vi "dfd_One Point Notch Peak Filter Design.vi"(7 "filter type":enum16{"Notch", "Peak"}(ring), 9 "normalized BW":dbl format="%.2f", 10 "Ab [dB]":dbl format="%.2f", 11 "normalized f0":dbl format="%.2f") -> (1 "denominator":dbl[](array[numeric]) format="%.2f", 2 "numerator":dbl[](array[numeric]) format="%.2f")   [LabVIEW 2017, in "NI_DigFilter_Design.lvlib"]
uses:
  <vilib>/addons/Digital Filter Design/NI_DigFilter_Design.lvlib
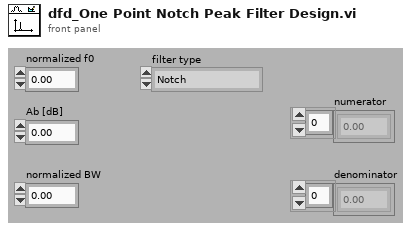
[diagram p1: front panel]
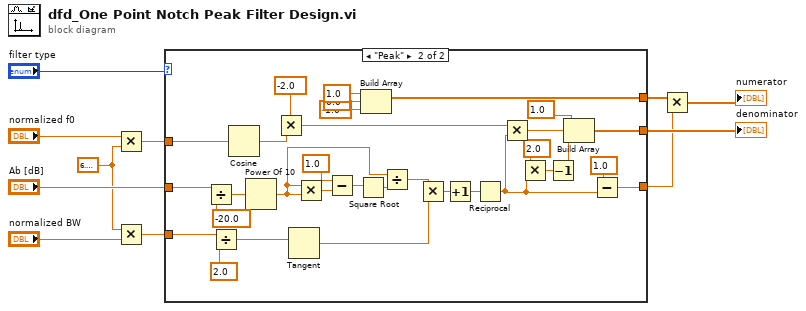
[diagram p0: block diagram]
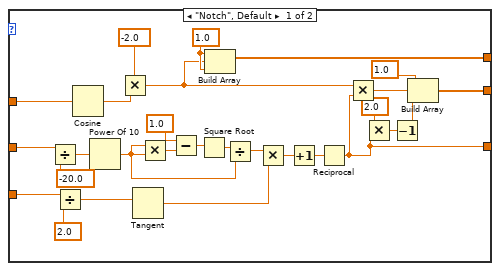
[diagram p2: hidden frame]
diagram:
  w3 = 6.283185307179586
  n1 = Multiply(x="normalized f0", y=w3) -> (x*y=w4:dbl)
  n2 = Multiply(x=w3, y="normalized BW") -> (x*y=w5:dbl)
  n3 = case shown="\"Peak\"" "filter type" {
    tunnel: "Ab [dB]" -> [w38 w70]
    tunnel: w5 -> [w34 w41]
    tunnel: [w21 w46] -> w6
    tunnel: w4 -> [w27 w40]
    tunnel: [w24 w60] -> w7
    tunnel: [w16 w54] -> w11
    frame "Notch", Default {
      w28 = 1.0 ("element")
      n4 = Divide(x=w38, y=-20.0) -> (x/y=w33:dbl)
      n5 = Divide(x=w34, y=2.0) -> (x/y=w29:dbl)
      n6 = Cosine(x=w27) -> (cos(x)=w26:dbl)
      n7 = Power Of 10(x=w33) -> (10^x=w35:dbl)
      n8 = Multiply(x=-2.0, y=w26) -> (x*y=w23:dbl)
      n9 = Tangent(1:w29) -> (0:w12:dbl)
      n10 = Multiply(x=w35, y=w35) -> (x*y=w37:dbl)
      n11 = Subtract(x=1.0, y=w37) -> (x-y=w15:dbl)
      n12 = Square Root(x=w15) -> (sqrt(x)=w14:dbl)
      n13 = Build Array(w28, w23, w28) -> (w24:dbl[])
      n14 = Divide(x=w14, y=w35) -> (x/y=w13:dbl)
      n15 = Multiply(x=w13, y=w12) -> (x*y=w31:dbl)
      n16 = Increment(x=w31) -> (x+1=w30:dbl)
      n17 = Reciprocal(x=w30) -> (1/x=w21:dbl)
      n18 = Multiply(x=w23, y=w21) -> (x*y=w22:dbl)
      n19 = Multiply(x=2.0 ("y"), y=w21) -> (x*y=w19:dbl)
      n20 = Decrement(x=w19) -> (x-1=w18:dbl)
      n21 = Build Array(1.0 ("element"), w22, w18) -> (w16:dbl[])
    }
    frame "Peak" {
      n22 = Divide(x=w70, y=-20.0) -> (x/y=w67:dbl)
      n23 = Divide(x=w41, y=2.0) -> (x/y=w63:dbl)
      n24 = Cosine(x=w40) -> (cos(x)=w62:dbl)
      n25 = Power Of 10(x=w67) -> (10^x=w53:dbl)
      n26 = Multiply(x=-2.0, y=w62) -> (x*y=w45:dbl)
      n27 = Tangent(1:w63) -> (0:w49:dbl)
      n28 = Multiply(x=w53, y=w53) -> (x*y=w69:dbl)
      n29 = Subtract(x=1.0, y=w69) -> (x-y=w52:dbl)
      n30 = Square Root(x=w52) -> (sqrt(x)=w51:dbl)
      n31 = Build Array(1.0 ("element"), 0.0 ("element"), -1.0 ("element")) -> (w60:dbl[])
      n32 = Divide(x=w53, y=w51) -> (x/y=w50:dbl)
      n33 = Multiply(x=w50, y=w49) -> (x*y=w65:dbl)
      n34 = Increment(x=w65) -> (x+1=w64:dbl)
      n35 = Reciprocal(x=w64) -> (1/x=w47:dbl)
      n36 = Multiply(x=w45, y=w47) -> (x*y=w59:dbl)
      n37 = Multiply(x=2.0 ("y"), y=w47) -> (x*y=w57:dbl)
      n38 = Decrement(x=w57) -> (x-1=w56:dbl)
      n39 = Build Array(1.0 ("element"), w59, w56) -> (w54:dbl[])
      n40 = Subtract(x=1.0, y=w47) -> (x-y=w46:dbl)
    }
  }
  "denominator" <- w11
  n41 = Multiply(x=w7, y=w6) -> (x*y=→"numerator":dbl[])
